vi "Test 622-182.vi"() -> ()   [LabVIEW 2021]
uses:
  Controls/Stepper Config.ctl
  Keithley 622x2182 Driver.lvclass
  C:/GitHub/NHMFL_Core/Libraries/Instruments/VISA Instrument/VISA Instrument.lvclass
  VISA Instrument/VISA Instrument.lvclass/VISA Instrument.ctl
  Results/Combined Result/Combined Result.lvclass
  VISA Instrument/Write VISA resource.vi
  Results/Acquired Result/Acquired Result.lvclass
panel:
  in  "Stop Button":bool
  out "Wait cycles":i32
  out "index":i32
  out "Waveform Graph 3":waveform(dbl)(graph)
  out "Waveform Graph 2":waveform(dbl)(graph)
  in  "Repeat":i32=1
  out "Waveform Graph":waveform(dbl)(graph)
  out "Availiable Samples":u32
  in  "Scan Configuration":T1={"Start"=-0.0001, "End"=0.0001, "Step"=1e-05, "Delta"=1e-05, "Scan shape"=enum."Sawtooth", "Append measurements"=[], "Pulse duration"=0.01, "Step duration"=0.2, "Scan mode"=enum."Diff. conductance"} {"Step duration" format="%#_6ps"; "Pulse duration" format="%#_6ps"; "Delta" format="%#_6p"; "Step" format="%#_6p"; "End" format="%#_6p"; "Start" format="%#_6p"}
  in  "VISA resource name":refnum<visa-resource-name>="GPIB0::1::INSTR"
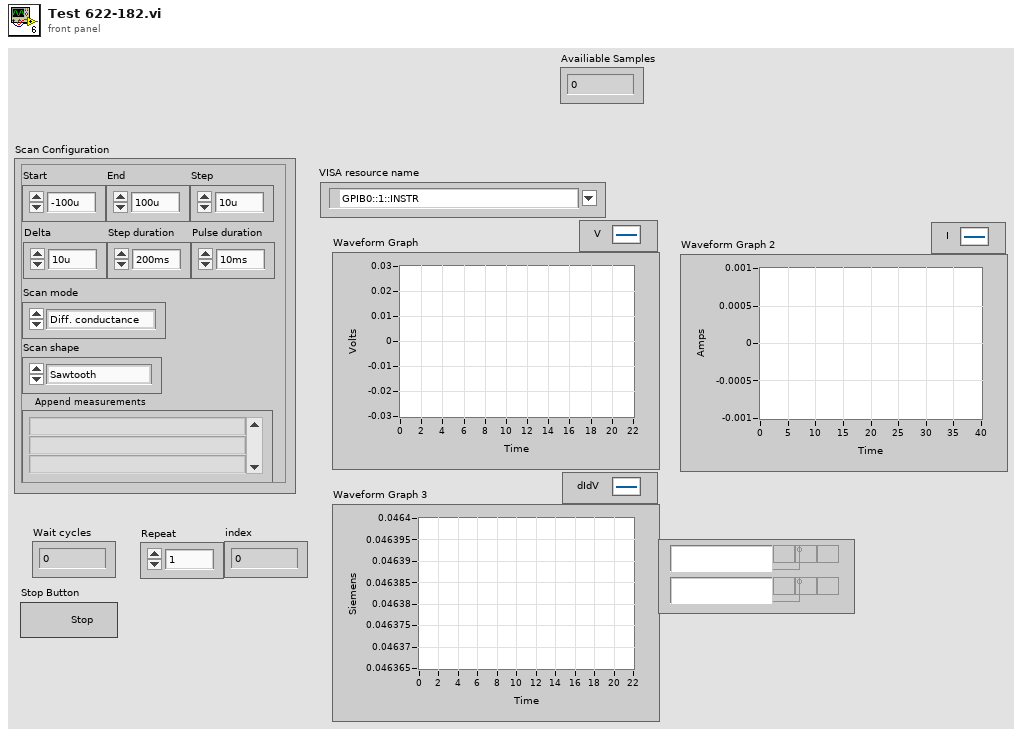
[diagram p1: front panel]
types:
  T1 = typedef "Stepper Config.ctl" = cluster{"Start":dbl, "End":dbl, "Step":dbl, "Delta":dbl, "Scan shape":enum16{"Sawtooth", "Triangular"}, "Append measurements":string[], "Pulse duration":dbl, "Step duration":dbl, "Scan mode":enum16{"Diff. conductance", "Pulse delta sweep"}}
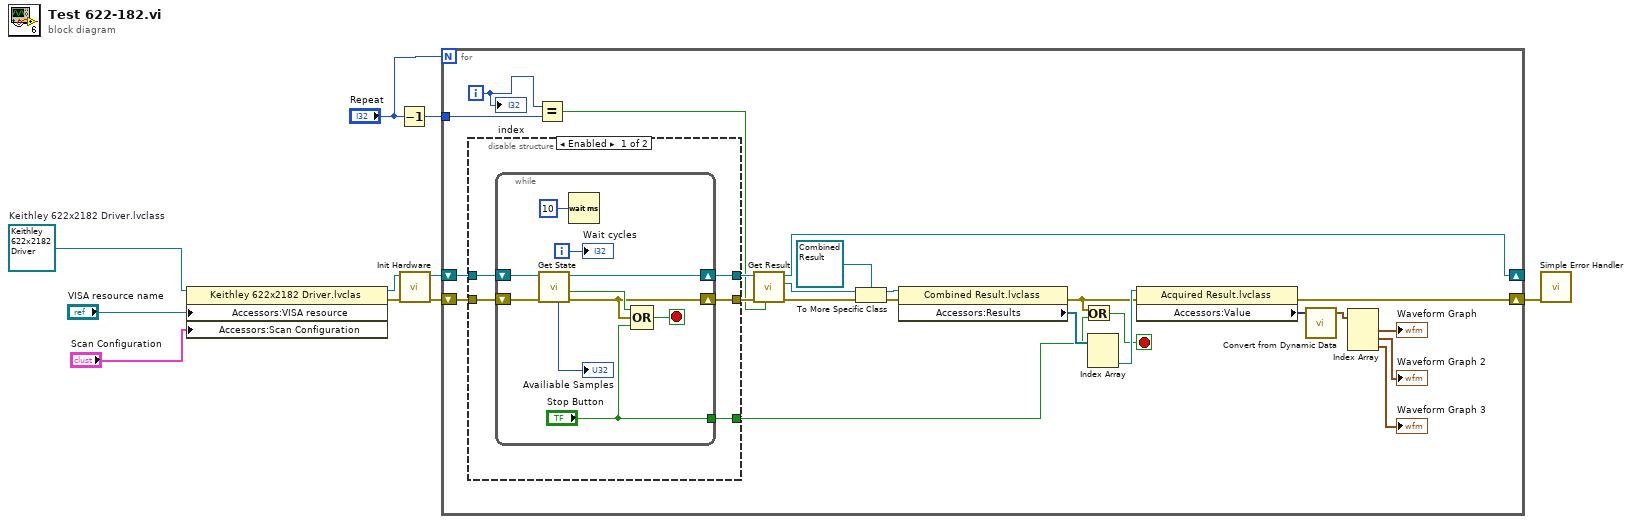
[diagram p0: block diagram]
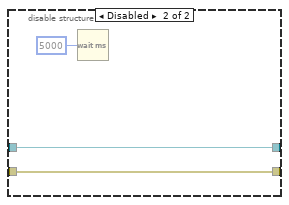
[diagram p2: hidden frame]
diagram:
  w10 = refnum<class "Keithley 622x2182 Driver.lvclass"> refnum  # Keithley 622x2182 Driver.lvclass
  n1 = property class="Keithley 622x2182 Driver.lvclas"(reference=w10, "Accessors:VISA resource"="VISA resource name", "Accessors:Scan Configuration"="Scan Configuration") -> (reference out=w8:refnum<class "Keithley 622x2182 Driver.lvclass">, error out=w7:errorcluster)  [unwired: 1 in]
  n2 = Decrement(x="Repeat") -> (x-1=w1:i32)
  n3 = call-dynamic "Init Hardware.vi"("error in (no error)"=w7, "Keithley 622x Driver in"=w8) -> ("error out"=w6:errorcluster, "Keithley 622x Driver out"=w5:refnum<class "Keithley 622x2182 Driver.lvclass">)  [unwired: 8 in]
  n4 = for {
    N: "Repeat" -> [_]
    shift-right: [w16] -> w4
    shift-left: w6 -> [w34]
    shift-right: [w30] -> _
    shift-left: w5 -> [w33]
    tunnel: w1 -> [w14]
    i -> [w15]
    stop <- w12 stop-if-true
    n5 = disable-structure shown="Enabled" {
      disable-tunnel: w34 -> [w39 w51]
      disable-tunnel: w33 -> [w38 w52]
      disable-tunnel: [w37 w52] -> w32
      disable-tunnel: [w36 w51] -> w31
      disable-tunnel: [w35 _] -> w11
      frame Enabled {
        n6 = while {
          shift-right: [w47] -> w37
          shift-left: w38 -> [w49]
          shift-right: [w42] -> w36
          shift-left: w39 -> [w48]
          tunnel: ["Stop Button"] -> w35
          i -> [w41]
          stop <- w44 stop-if-true
          n7 = call-dynamic "Get State.vi"("error in (no error)"=w48, "Keithley 622x2182 Driver in"=w49) -> ("error out"=w42:errorcluster, "Data ready"=w43:bool, "Keithley 622x2182 Driver out"=w47:refnum<class "Keithley 622x2182 Driver.lvclass">, "Availiable Samples"=→"Availiable Samples":u32)  [unwired: 4 in, 2 out]
          n8 = Wait (ms)(milliseconds to wait=u32 10) -> ()  [unwired: 1 out]
          n9 = Compound Arithmetic op=OR(w43, w42, "Stop Button") -> (w44:bool)
          "Wait cycles" <- w41
        }
      }
      frame Disabled {
        n10 = Wait (ms)(milliseconds to wait=u32 5000) -> ()  [unwired: 1 out]
      }
    }
    n11 = Equal?(x=w15, y=w14) -> (x = y?=w13:bool)
    n12 = call-dynamic "Get Result.vi"("Last request"=w13, "error in (no error)"=w31, "Keithley 622x2182 Driver in"=w32) -> ("error out"=w29:errorcluster, "Result"=w24:refnum<class "Acquired Result.lvclass">, "Keithley 622x2182 Driver out"=w30:refnum<class "Keithley 622x2182 Driver.lvclass">)  [unwired: 6 in]
    n13 = To More Specific Class(target class=refnum<class "Combined Result.lvclass"> refnum ("Combined Result.lvclass"), reference=w24, error in=w29) -> (specific class reference=w23:refnum<class "Combined Result.lvclass">, error out=w25:errorcluster)
    n14 = property class="Combined Result.lvclass"(reference=w23, error in=w25) -> (error out=w17:errorcluster, "Accessors:Results"=w21:refnum<class "Acquired Result.lvclass">[])  [unwired: 1 out]
    n15 = Or(x=w17, y=w11) -> (x .or. y?=w12:bool)
    n16 = Index Array(array=w21) -> (element #2=w20:refnum<class "Acquired Result.lvclass">)  [unwired: 2 in, 1 out]
    n17 = property class="Acquired Result.lvclass"(reference=w20, error in=w17) -> (error out=w16:errorcluster, "Accessors:Value"=w19:dynamicdata)  [unwired: 1 out]
    n18 = call "Convert from Dynamic Data"("Dynamic Data Type"=w19) -> ("Array of Waveform"=w18:waveform(dbl)[])  [unwired: 3 in]
    n19 = Index Array(array=w18) -> (element #1=→"Waveform Graph":waveform(dbl), element #2=→"Waveform Graph 2":waveform(dbl), element #3=→"Waveform Graph 3":waveform(dbl))  [unwired: 3 in]
    "index" <- w15
  }
  n20 = call <vilib>:"Simple Error Handler.vi"("error in (no error)"=w4) -> ()  [unwired: 4 in, 5 out]
